vi "SPI Master.vi"(5 "Count":u16, 7 "Configuration":u16 format="%016b", 8 "Start?":T1, 10 "MISO":bool, 11 "Data Out":u16) -> (0 "Status":u8 format="%08b", 1 "SCLK":bool, 2 "MOSI":bool, 3 "Data In":u16)   [LabVIEW 2017]
doc: "This VI handles the SPI protocol to transfer data between master and slave devices using <b>MISO </b>(Master In Slave Out), <b>MOSI </b>(Master Out Slave In), and <b>SCLK </b>(Serial Clock)."
uses:
  Utilities/Start Boolean.ctl
  SPI States.ctl
  SPI Frame Length.ctl
panel:
  # "This VI handles the SPI protocol to transfer data between master and slave devices using MISO (Master In Slave Out), MOSI (Master Out Slave In), and SCLK (Serial Clock).\n \nSPI Configuration:                         SPI Status:\nBit [15:14] : Clock Select                Bit [7:1]  : Reserved\nBit [13:8]   : Reseved                       Bit 0        : SPI subsystem is Busy\nBit [7:4]     : Frame Length\nBit 3           : Data Order\nBit 2           : Clock Polarity\nBit 1           : Clock Phase\nBit 0       : Reserved"
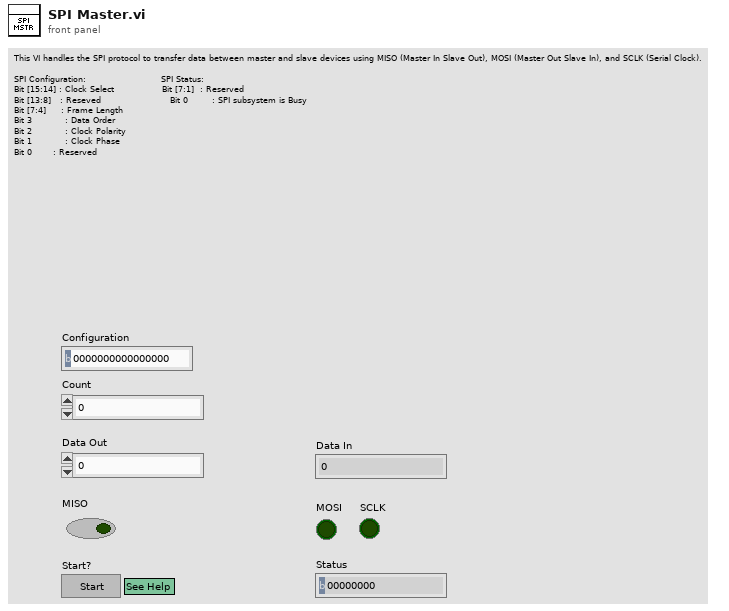
[diagram p1: front panel]
types:
  T1 = typedef "Start Boolean.ctl" = bool
  T2 = typedef "SPI Frame Length.ctl" = fxp<+,4,4>
  T3 = typedef "SPI States.ctl" = fxp<+,3,3>
  T4 = typedef "SPI Clock Select.ctl" = fxp<+,2,2>
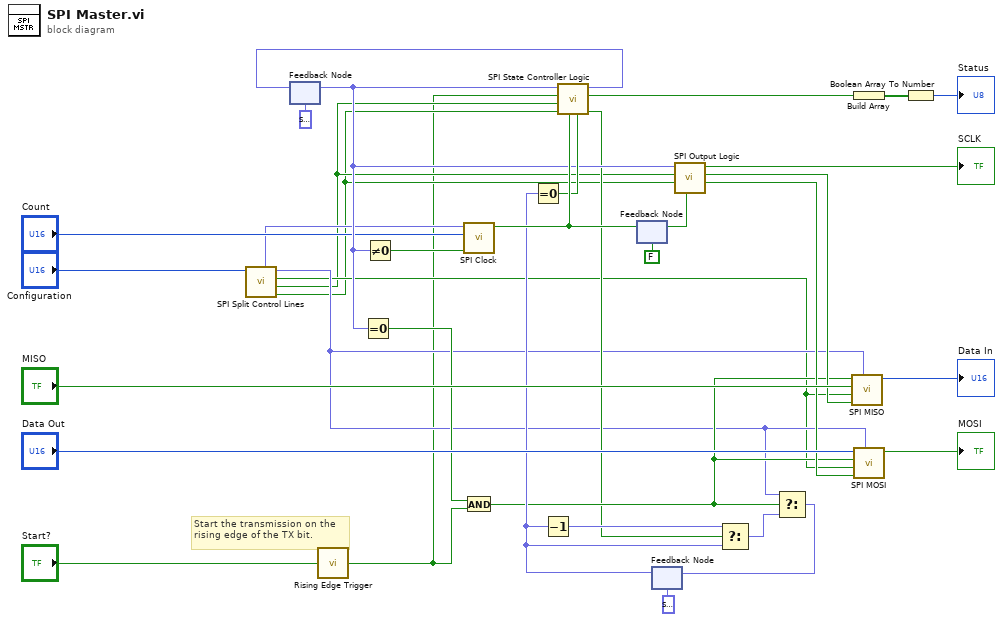
[diagram p0: block diagram]
diagram:
  # "Start the transmission on the rising edge of the TX bit."
  n1 = call "SPI Split Control Lines.vi"("SPCR"="Configuration") -> ("Sample on trailing edge (Phase)?"=w7:bool, "Falling edge leads (Polarity)?"=w8:bool, "LSB first?"=w9:bool, "Frame Length"=w10:T2, "Clock Select"=w11:T4)  [unwired: 5 in, 1 out]
  n2 = feedback #1(T3 0.0 ("State+")) -> (w17:T3)
  n3 = call "Rising Edge Trigger.vi"("Signal"="Start?") -> ("Trigger?"=w3:bool)
  n4 = Equal To 0?(x=w17) -> (x = 0?=w20:bool)
  n5 = Not Equal To 0?(x=w17) -> (x != 0?=w6:bool)
  n6 = call "SPI Clock.vi"("Count?"=w6, "Max Value"="Count", "Clock Select"=w11) -> ("Enable Out"=w29:bool)  [unwired: 8 in]
  n7 = And(x=w20, y=w3) -> (x .and. y?=w21:bool)
  n8 = feedback #2(FALSE ("Enable Out")) -> (w28:bool)
  n9 = feedback-in #2(w29) -> ()
  n10 = feedback #3(T2 0.0) -> (w22:T2)
  n11 = Equal To 0?(x=w22) -> (x = 0?=w19:bool)
  n12 = Decrement(x=w22) -> (x-1=w23:T2)
  n13 = call "SPI State Controller Logic.vi"("Frame Complete?"=w19, "Enable?"=w29, "Sample on trailing edge (Phase)?"=w7, "Falling edge leads (Polarity)?"=w8, "Start?"=w3, "State"=w17) -> ("Increment?"=w14:bool, "Busy?"=w1:bool, "State+"=w18:T3)  [unwired: 3 in]
  n14 = feedback-in #1(w18) -> ()
  n15 = call "SPI Output Logic.vi"("Enable?"=w28, "Sample on trailing edge (Phase)?"=w7, "Falling edge leads (Polarity)?"=w8, "State"=w17) -> ("Setup?"=w30:bool, "Sample?"=w31:bool, "SCLK"=→"SCLK":bool)  [unwired: 4 in, 1 out]
  n16 = Select(t=w23, s=w14, f=w22) -> (s? t:f=w25:T2)
  n17 = Select(t=w10, s=w21, f=w25) -> (s? t:f=w24:T2)
  n18 = feedback-in #3(w24) -> ()
  n19 = call "SPI MISO.vi"("Index"=w10, "Sample?"=w31, "LSB first?"=w9, "MISO"="MISO", "Reset?"=w21) -> ("Data In"=→"Data In":u16)  [unwired: 6 in]
  n20 = Build Array(w1) -> (w5:bool[])
  n21 = call "SPI MOSI.vi"("Index"=w10, "Setup?"=w30, "LSB first?"=w9, "Load?"=w21, "Data Out"="Data Out") -> ("MOSI"=→"MOSI":bool)  [unwired: 6 in]
  n22 = Boolean Array To Number(Boolean array=w5) -> (number=→"Status":u8)
